vi "Error source chain.vi"(7 "Generate message (T)":bool=TRUE, 8 "error in (no error)":errorcluster, 9 "Skip levels(0)":u32, 10 "Explanation":string, 11 "New Error Code":i32=-2147483648) -> (0 "error out":errorcluster)   [LabVIEW 2009]
doc: "Sets the error source to the concat of the Explanation and the call chain in case of an error. This error may allready be present in the error cluster or in the new error code. Skip levels is the number of low level vi's that are not to be mentioned in the call chain. Value 0 skips only this vi."
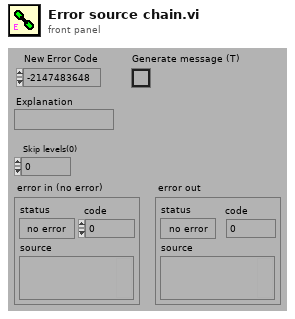
[diagram p1: front panel]
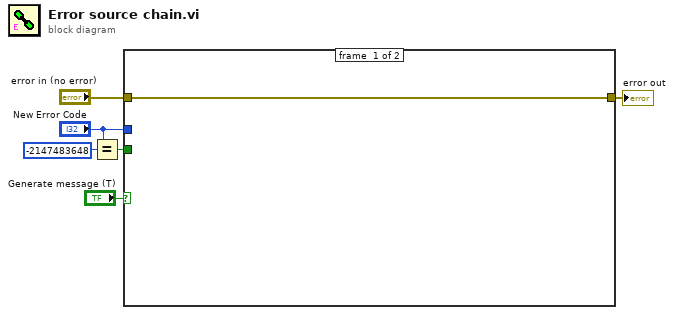
[diagram p0: block diagram]
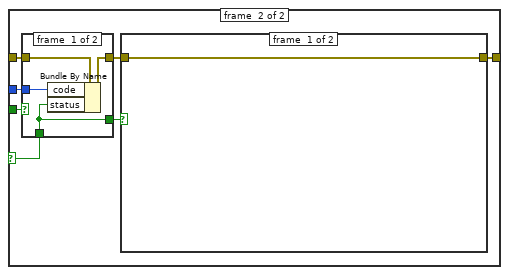
[diagram p2: hidden frame]
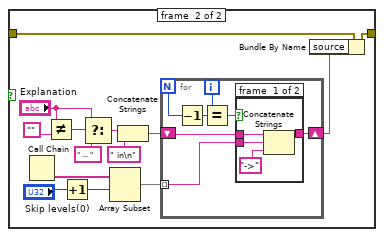
[diagram p3: hidden frame]
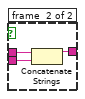
[diagram p4: hidden frame]
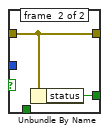
[diagram p5: hidden frame]
diagram:
  n1 = Equal?(x=-2147483648, y="New Error Code") -> (x = y?=w5:bool)
  n2 = case shown="True" "Generate message (T)" {
    selector: "Generate message (T)" -> [_ w8]
    tunnel: "error in (no error)" -> [w7 w12]
    tunnel: "New Error Code" -> [_ w11]
    tunnel: w5 -> [_ w10]
    tunnel: [w7 w9] -> w6
    frame #0 {
    }
    frame #1 {
      n3 = case shown="True" w10 {
        tunnel: [w47 w49] -> w13
        tunnel: w12 -> [w46 w49]
        tunnel: w11 -> [w45 _]
        tunnel: [w44 w48] -> w14
        tunnel: w8 -> [w44 _]
        frame #0 {
          n4 = Bundle By Name(cluster=w46, "code"=w45, "status"=w44) -> (w47:errorcluster)
        }
        frame #1 {
          n5 = Unbundle By Name(w49) -> ("status"=w48:bool)
        }
      }
      n6 = case shown="True" w14 {
        tunnel: w13 -> [w15 w17]
        tunnel: [w15 w29] -> w9
        frame #0 {
        }
        frame #1 {
          n7 = Call Chain() -> (call chain=w27:string[])
          n8 = Not Equal?(x="Explanation", y="") -> (x != y?=w22:bool)
          n9 = Increment(x="Skip levels(0)") -> (x+1=w25:u32)
          n10 = Select(t="Explanation", s=w22, f=" ... ") -> (s? t:f=w20:string)
          n11 = Array Subset(array=w27, index=w25) -> (w28:string[])  [unwired: 1 in]
          n12 = Concatenate Strings(w20, " in\n") -> (w18:string)
          n13 = for {
            N -> [w36]
            tunnel: w28 -> [w31] mode=indexing
            shift-right: [w32] -> w16
            shift-left: w18 -> [w33]
            i -> [w34]
            n14 = Decrement(x=w36) -> (x-1=w35:i32)
            n15 = Equal?(x=w35, y=w34) -> (x = y?=w30:bool)
            n16 = case shown="False" w30 {
              tunnel: w31 -> [w39 w43]
              tunnel: [w38 w42] -> w32
              tunnel: w33 -> [w37 w41]
              frame #0 {
                n17 = Concatenate Strings(w37, w39, "->") -> (w38:string)
              }
              frame #1 {
                n18 = Concatenate Strings(w41, w43) -> (w42:string)
              }
            }
          }
          n19 = Bundle By Name(cluster=w17, "source"=w16) -> (w29:errorcluster)
        }
      }
    }
  }
  "error out" <- w6
